vi "create_NewHost.vi"() -> (14 "MoAgSy_Host.lvclass out":refnum<class "MoAgSy_Host.lvclass">, 16 "Cancel":bool, 19 "error out":errorcluster)   [LabVIEW 2009, in "MoAgSy.lvlib" / "MoAgSy_Host.lvclass"]
doc: "<B>public</B> VI.\nGUI to initiate a new Host.\nUser input:\nGeneral settings (host name, max number of running agents)\nDirectory settings (local folder, local class folder)\nFTP settings (FTP host, FTP username, FTP password, remote port, load libs)\n\nF.Berck@gsi.de\nGSI Darmstadt 2009"
uses:
  MoAgSy_Host.lvclass
  MoAgSy_GPG/MoAgSy_GPG.lvclass
  MoAgSy_Factory/MoAgSy_Factory.lvclass
  MoAgSy_Host.lvclass/MoAgSy_Host.ctl
  HGF_BaseClasses/HGF_Factory/HGF_Factory.lvclass
  MoAgSy.lvlib
panel:
  in  "General Settings":T1
  in  "Previous":bool
  in  "Cancel":bool
  in  "FTP Settings":T2={"FTP Host"="", "FTP Username"="", "FTP Password"="", "remote port (21)"=21, "Load new libs from FTP server"=FALSE}
  in  "Next":bool
  in  "Set Directories":T3
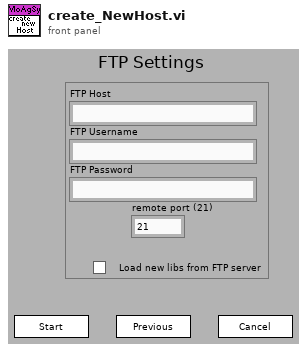
[diagram p1: front panel]
types:
  T1 = cluster{"Host ID":string, "Maximum number of running Agents":i16}
  T2 = cluster{"FTP Host":string, "FTP Username":string, "FTP Password":string, "remote port (21)":u16, "Load new libs from FTP server":bool}
  T3 = cluster{"Working Folder":path, "Class Folder":path}
  T4 = cluster{"Host Name":string, "Maximum Nof running Agents":i16, "ID":string}
  T5 = enum16{"Directories", "General Settings", "FTP Settings", "End"}
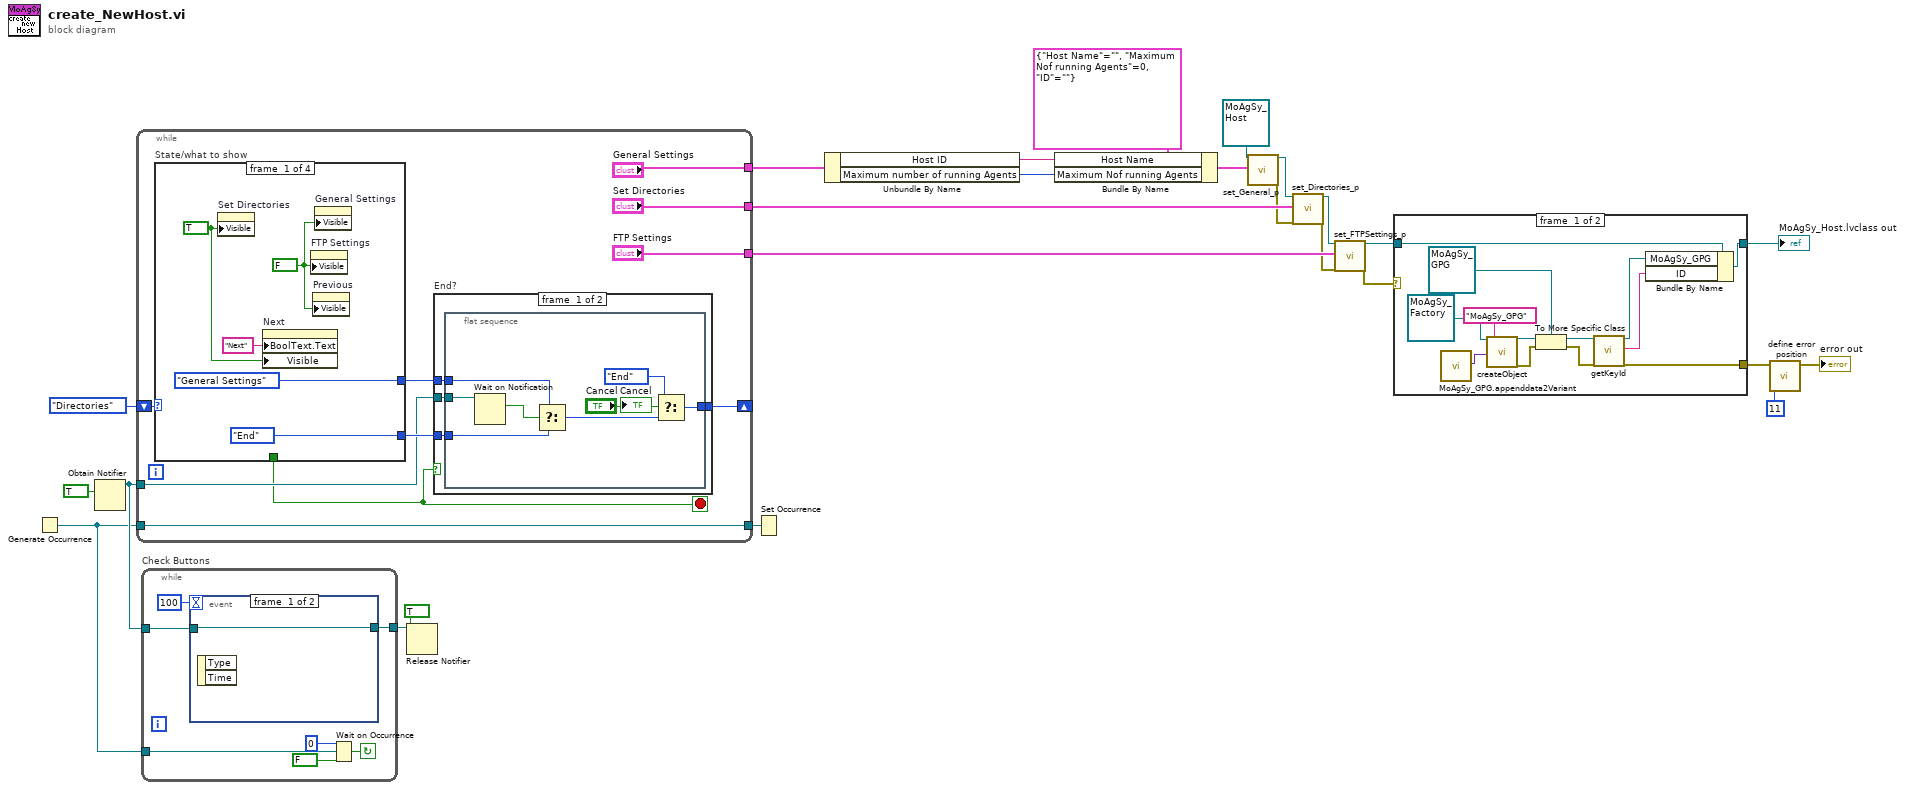
[diagram p0: block diagram]
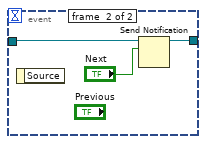
[diagram p3: hidden frame]
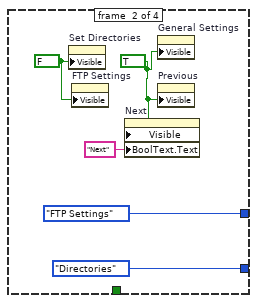
[diagram p5: hidden frame]
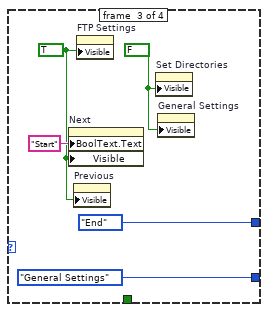
[diagram p6: hidden frame]
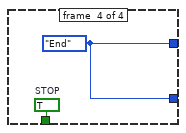
[diagram p7: hidden frame]
diagram:
  n1 = Generate Occurrence() -> (w12:refnum<k4>)
  n2 = Obtain Notifier(notification data type=TRUE) -> (notifier out=w21:refnum<notifier>)  [unwired: 2 in, 3 out]
  n3 = while {
    shift-right: [w32] -> _
    shift-left: T5."Directories" ("Enum") -> [w35]
    tunnel: w21 -> [w31]
    tunnel: ["Set Directories"] -> w20
    tunnel: ["General Settings"] -> w3
    tunnel: ["FTP Settings"] -> w19
    tunnel: w12 -> [w28]
    tunnel: [w28] -> w13
    stop <- w27 stop-if-true
    n4 = case "State/what to show" shown="\"End\"" w35 {
      tunnel: [_ _ _ w64] -> w27
      tunnel: [T5."General Settings" ("Enum") T5."FTP Settings" ("Enum") T5."End" ("Enum") w63] -> w34
      tunnel: [T5."End" ("Enum") T5."Directories" ("Enum") T5."General Settings" ("Enum") w63] -> w33
      frame #0 {
        w48 = FALSE ("Visible")
        w49 = TRUE ("Visible")
        n5 = property on="Set Directories" class="Clust (strict)"("Visible"=w49) -> ()  [unwired: 2 in, 2 out]
        n6 = property on="Next" class="Bool"("BoolText.Text"="Next" ("Boolean Text.Text"), "Visible"=w49) -> ()  [unwired: 2 in, 2 out]
        n7 = property on="FTP Settings" class="Clust (strict)"("Visible"=w48) -> ()  [unwired: 2 in, 2 out]
        n8 = property on="Previous" class="Bool"("Visible"=w48) -> ()  [unwired: 2 in, 2 out]
        n9 = property on="General Settings" class="Clust (strict)"("Visible"=w48) -> ()  [unwired: 2 in, 2 out]
      }
      frame #1 {
        w53 = TRUE ("Visible")
        w54 = FALSE ("Visible")
        n10 = property on="Set Directories" class="Clust (strict)"("Visible"=w54) -> ()  [unwired: 2 in, 2 out]
        n11 = property on="FTP Settings" class="Clust (strict)"("Visible"=w54) -> ()  [unwired: 2 in, 2 out]
        n12 = property on="Next" class="Bool"("Visible"=w53, "BoolText.Text"="Next" ("Boolean Text.Text")) -> ()  [unwired: 2 in, 2 out]
        n13 = property on="General Settings" class="Clust (strict)"("Visible"=w53) -> ()  [unwired: 2 in, 2 out]
        n14 = property on="Previous" class="Bool"("Visible"=w53) -> ()  [unwired: 2 in, 2 out]
      }
      frame #2 {
        w58 = FALSE ("Visible")
        w59 = TRUE ("Visible")
        n15 = property on="Next" class="Bool"("BoolText.Text"="Start" ("Boolean Text.Text"), "Visible"=w59) -> ()  [unwired: 2 in, 2 out]
        n16 = property on="Previous" class="Bool"("Visible"=w59) -> ()  [unwired: 2 in, 2 out]
        n17 = property on="FTP Settings" class="Clust (strict)"("Visible"=w59) -> ()  [unwired: 2 in, 2 out]
        n18 = property on="Set Directories" class="Clust (strict)"("Visible"=w58) -> ()  [unwired: 2 in, 2 out]
        n19 = property on="General Settings" class="Clust (strict)"("Visible"=w58) -> ()  [unwired: 2 in, 2 out]
      }
      frame #3 {
        w63 = T5."End" ("Enum")
        w64 = TRUE  # STOP
      }
    }
    n20 = case "End?" shown="False" w27 {
      tunnel: w34 -> [w39 _]
      tunnel: w33 -> [w38 _]
      tunnel: [w37 _] -> w32
      tunnel: w31 -> [w36 _]
      frame #0 {
        n21 = flat-sequence {
          tunnel: w39 -> [w47]
          tunnel: w38 -> [w46]
          tunnel: [w43] -> w37
          tunnel: w36 -> [w42]
          frame #0 {
            n22 = Wait on Notification(notifier=w42) -> (notification=w41:bool)  [unwired: 1 in, 5 out]
            n23 = Select(t=w47, s=w41, f=w46) -> (s? t:f=w44:T5)
            n24 = Select(t=T5."End" ("Enum"), s="Cancel", f=w44) -> (s? t:f=w43:T5)
            "Cancel" <- "Cancel"
          }
        }
      }
      frame #1 {
      }
    }
  }
  n25 = while "Check Buttons" {
    tunnel: w21 -> [w70]
    tunnel: [w69] -> w23
    tunnel: w12 -> [w68]
    stop <- w65 continue-if-true
    n26 = event shown="[1] \"Previous\", \"Cancel\", \"Next\": Value Change" {
      selector: _ -> [_ _]
      dyn-events: _ -> [_ _]
      timeout: 100 -> [_ _]
      tunnel: w70 -> [w72 w75]
      tunnel: [w72 w73] -> w69
      event #0 {
        n27 = event-data() -> ()  [unwired: 3 out]
      }
      event #1 {
        n28 = event-data() -> ()  [unwired: 2 out]
        n29 = Send Notification(notification="Next", notifier=w75) -> (notifier out=w73:refnum<notifier>)  [unwired: 1 in, 1 out]
      }
    }
    n30 = Wait on Occurrence(1:FALSE ("ignore previous (T)"), 2:w68, 3:0 ("ms timeout (-1)")) -> (0:w65:bool)
  }
  n31 = Release Notifier(notifier=w23, force destroy? (F)=TRUE) -> ()  [unwired: 1 in, 3 out]
  n32 = Set Occurrence(w13) -> ()
  n33 = Unbundle By Name(w3) -> ("Host ID"=w2:string, "Maximum number of running Agents"=w1:i16)
  n34 = Bundle By Name(cluster=T4 {"Host Name"="", "Maximum Nof running Agents"=0, "ID"=""} ("General"), "Host Name"=w2, "Maximum Nof running Agents"=w1) -> (w4:T4)
  n35 = call "set_General_p.vi"("MoAgSy_Host"=refnum<class "MoAgSy_Host.lvclass"> refnum ("MoAgSy.lvlib:MoAgSy_Host.lvclass"), "General"=w4) -> ("dup MoAgSy_Host"=w17:refnum<class "MoAgSy_Host.lvclass">, "error out"=w14:errorcluster)  [unwired: 1 in, 15 out]
  n36 = call "set_Directories_p.vi"("MoAgSy_Host"=w17, "Directories"=w20, "error in (no error)"=w14) -> ("dup MoAgSy_Host"=w16:refnum<class "MoAgSy_Host.lvclass">, "error out"=w15:errorcluster)  [unwired: 15 out]
  n37 = call "set_FTPSettings_p.vi"("MoAgSy_Host"=w16, "FTP Settings"=w19, "error in (no error)"=w15) -> ("dup MoAgSy_Host"=w10:refnum<class "MoAgSy_Host.lvclass">, "error out"=w11:errorcluster)  [unwired: 15 out]
  n38 = case shown="No Error" w11 {
    selector: w11 -> [_ w89]
    tunnel: [w77 w89] -> w8
    tunnel: w10 -> [w82 w90]
    tunnel: [w81 w90] -> w9
    frame #0 {
      n39 = call "MoAgSy_GPG.appenddata2Variant.vi"() -> ("dup initData"=w84:variant)  [unwired: 1 in, 18 out]
      n40 = call "createObject.vi"("HGF_Factory"=refnum<class "MoAgSy_Factory.lvclass"> refnum ("MoAgSy.lvlib:MoAgSy_Factory.lvclass"), "initializationData"=w84, "className"="MoAgSy_GPG") -> ("HGF_Object"=w86:refnum<class "HGF_Factory.lvclass">, "error out"=w88:errorcluster)  [unwired: 2 in, 13 out]
      n41 = To More Specific Class(target class=refnum<class "MoAgSy_GPG.lvclass"> refnum ("MoAgSy.lvlib:MoAgSy_GPG.lvclass"), reference=w86, error in=w88) -> (specific class reference=w80:refnum<class "MoAgSy_GPG.lvclass">, error out=w78:errorcluster)
      n42 = call-dynamic "getKeyId.vi"("HGF_GPG.lvclass in"=w80, "error in (no error)"=w78) -> ("HGF_GPG.lvclass out"=w79:refnum<class "MoAgSy_GPG.lvclass">, "Key-ID"=w76:string, "error out"=w77:errorcluster)  [unwired: 15 in]
      n43 = Bundle By Name(cluster=w82, "MoAgSy_GPG"=w79, "ID"=w76) -> (w81:refnum<class "MoAgSy_Host.lvclass">)
    }
    frame #1 {
    }
  }
  "MoAgSy_Host.lvclass out" <- w9
  n44 = call "define error position.vi"("Position"=11, "error in (no error)"=w8) -> ("error out"=→"error out":errorcluster)  [unwired: 8 in, 1 out]
